vi "Set DAC Output.vi"(9 "iValue":i32, 10 "iResolution":i32, 11 "iOption":i32) -> (3 "function return":u32)   [LabVIEW 2018, in "Copy of Andor SDK.lvlib"]
doc: "EXPNETTYPE unsigned int WINAPI SetDACOutput(int iOption, int iResolution, int iValue);"
uses:
  Copy of Andor SDK.lvlib
  <userlib>/Andor SDK/ATMCD32D.dll
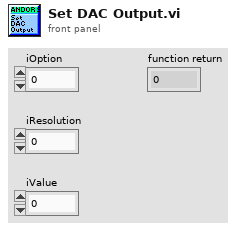
[diagram p1: front panel]
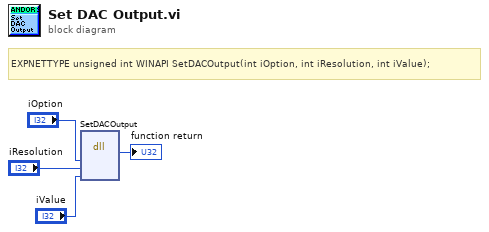
[diagram p0: block diagram]
diagram:
  # "EXPNETTYPE unsigned int WINAPI SetDACOutput(int iOption, int iResolution, int iValue);"
  n1 = dll-call lib="C:/Program Files (x86)/National Instruments/LabVIEW 2018/user.lib/Andor SDK/ATMCD32D.*" fn="SetDACOutput"("iOption"="iOption", "iResolution"="iResolution", "iValue"="iValue") -> (→"function return":u32)  [unwired: 6 in, 2 out]
